vi "Mat Write Test.vi"   [LabVIEW 2015]
uses:
  <userlib>/_matio/level5/Public/Write/Append Data Element.llb/Append Data Element (1D Array of Double).vi
  <userlib>/_matio/level5.lvlib
  <vilib>/Analysis/NI_AALBase.lvlib
types:
  T1 = enum16{"big-endian, network order", "native, host order", "little-endian"}
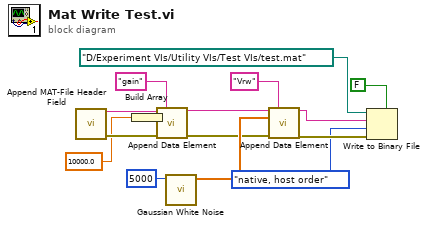
[diagram p0: block diagram]
diagram:
  n1 = call <userlib>:"Append MAT-File Header Field.vi"() -> ("result string"=w7:string, "error out"=w6:errorcluster)  [unwired: 14 in]
  n2 = Build Array(10000.0) -> (w1:dbl[])
  n3 = call-poly <userlib>:"Append Data Element.vi"("initial string"=w7, "Data Name"="gain", "data"=w1, "error in"=w6) -> ("result string"=w5:string, "error out"=w4:errorcluster)  [unwired: 10 in]
  n4 = call <vilib>:"Gaussian White Noise.vi"("samples"=5000) -> ("Gaussian noise pattern"=w14:dbl[])  [unwired: 9 in, 1 out]
  n5 = call-poly <userlib>:"Append Data Element.vi"("initial string"=w5, "Data Name"="Vrw", "data"=w14, "error in"=w4) -> ("result string"=w11:string, "error out"=w12:errorcluster)  [unwired: 10 in]
  n6 = Write to Binary File(file (use dialog)=path "D:/Experiment VIs/Utility VIs/Test VIs/test.mat", data=w11, error in=w12, 5:FALSE ("prepend array or string size? (T)"), 9:T1."native, host order" ("byte order (0:big-endian, network order)")) -> ()  [unwired: 1 in, 3 out]
